vi "Update Display.vi"(8 "error in (no error)":errorcluster, 11 "Game Engine in":refnum<class "Game Engine.lvclass">) -> (0 "error out":errorcluster, 3 "Game Engine out":refnum<class "Game Engine.lvclass">)   [LabVIEW 2017, in "Game Engine.lvlib" / "Game Engine.lvclass"]
uses:
  Game Engine.lvclass
  Game Engine.lvclass/Game Engine.ctl
  Screen Interface/Screen Interface Messages/Display Game Board Msg/Display Game Board Msg.lvclass/Display Game Board Msg.ctl
  <vilib>/ActorFramework/Message Enqueuer/Message Enqueuer.lvclass/Message Enqueuer.ctl
  <vilib>/ActorFramework/Message Enqueuer/Enqueue.vi
  Screen Interface/Screen Interface Messages/Display Game Board Msg/Display Game Board Msg.lvclass
  C:/Program Files (x86)/National Instruments/LabVIEW 2017/vi.lib/ActorFramework/Message/Message.lvclass
  <vilib>/ActorFramework/Message Priority Queue/Priority Enqueue.vi
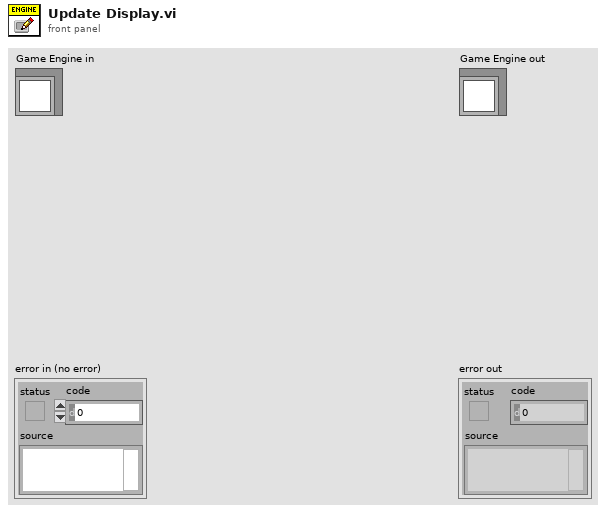
[diagram p1: front panel]
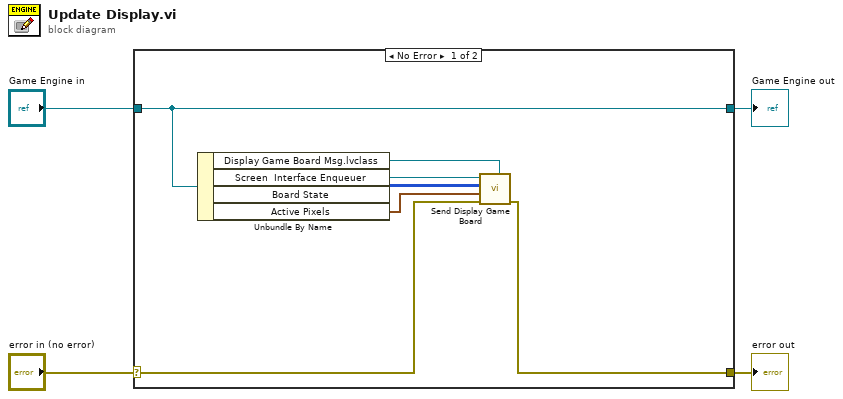
[diagram p0: block diagram]
diagram:
  n1 = case shown="No Error" "error in (no error)" {
    selector: "error in (no error)" -> [w7 w13]
    tunnel: [w6 w13] -> w3
    tunnel: [w11 w12] -> w1
    tunnel: "Game Engine in" -> [w11 w12]
    frame No Error {
      n2 = Unbundle By Name(w11) -> ("Display Game Board Msg.lvclass"=w5:refnum<class "Display Game Board Msg.lvclass">, "Screen  Interface Enqueuer"=w10:refnum<class "Message Enqueuer.lvclass">, "Board State"=w9:u32[][], "Active Pixels"=w8:cluster{"Column":u8, "Row":u8, "Color":u32}[])
      n3 = call "Send Display Game Board.vi"("Message Type"=w5, "error in (no error)"=w7, "Active Pixels"=w8, "Board State"=w9, "Message Enqueuer"=w10) -> ("error out"=w6:errorcluster)  [unwired: 5 in, 1 out]
    }
    frame Error {
    }
  }
  "error out" <- w3
  "Game Engine out" <- w1
